vi "API_Edit.vi"(1 "Cancel":bool, 2 "OK":bool, 3 "VI Path":path, 4 "Argument List In":string[](array[string])) -> (0 "Argument List Out":string[](array[string]))   [LabVIEW 2011]
doc: "This VI handles the event loop for API VI's in \"Edit Mode\". Note that the calling VI must have \"OK\" and \"Cancel\" buttons, with labels set as such. This VI also handles window modes for the calling API VI. This VI should always be used in conjunction with API_Init.vi.\n\nThe \"OK\" and \"Cancel\" parameters are optional. They are only necessary if the user wishes to implement their own edit mode event loop in the API VI. In this case, \"OK\" should be set to \"True\" if the user wishes to save the front panel controls in the \"Argument List\". Otherwise, \"Cancel\" should be set to \"True\". If neither of these parameters are set, this VI will handle the edit mode event loop itself."
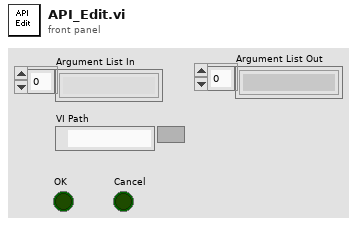
[diagram p1: front panel]
types:
  T1 = enum32{"Invalid", "Default", "Floating", "Floating/Auto-Hide", "Modal"}
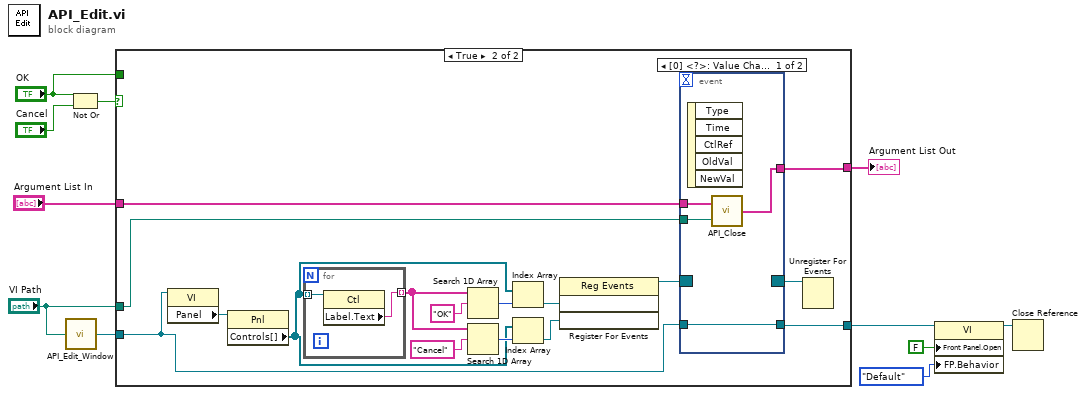
[diagram p0: block diagram]
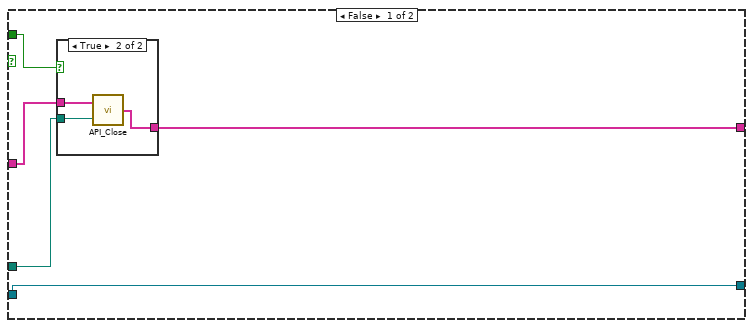
[diagram p2: hidden frame]
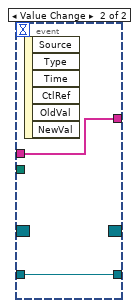
[diagram p4: hidden frame]
diagram:
  n1 = call "API_Edit_Window.vi"("VI Path"="VI Path") -> ("VI Reference"=w1:refnum<vi>)
  n2 = Not Or(1:"Cancel", 2:"OK") -> (0:w4:bool)
  n3 = case shown="True" w4 {
    tunnel: "Argument List In" -> [w14 w26]
    tunnel: "VI Path" -> [w13 w25]
    tunnel: [w12 w24] -> w9
    tunnel: [w16 w23] -> w8
    tunnel: w1 -> [w16 w21]
    tunnel: "OK" -> [w15 _]
    frame False {
      n4 = case shown="True" w15 {
        tunnel: w14 -> [w17 w20]
        tunnel: w13 -> [_ w19]
        tunnel: [w17 w18] -> w12
        frame False {
        }
        frame True {
          n5 = call "API_Close.vi"("VI Path"=w19, "Argument List In"=w20) -> ("Argument List Out"=w18:string[])
        }
      }
    }
    frame True {
      n6 = property class="VI"(reference=w21) -> ("Panel"=w36:refnum<vi>)  [unwired: 1 in, 2 out]
      n7 = property class="Pnl"(reference=w36) -> ("Controls[]"=w30:refnum<vi>[])  [unwired: 1 in, 2 out]
      n8 = for {
        tunnel: w30 -> [w44] mode=indexing
        tunnel: [w43] -> w33 mode=indexing
        n9 = property class="Ctl"(reference=w44) -> ("Label.Text"=w43:string)  [unwired: 1 in, 2 out]
      }
      n10 = Search 1D Array(1D array=w33, element="OK") -> (index of element=w32:i32)  [unwired: 1 in]
      n11 = Search 1D Array(1D array=w33, element="Cancel") -> (index of element=w31:i32)  [unwired: 1 in]
      n12 = Index Array(array=w30, index=w32) -> (element=w29:refnum<vi>)
      n13 = Index Array(array=w30, index=w31) -> (element=w27:refnum<vi>)
      n14 = register-events(w29, w27) -> (reference out=w28:refnum<event-registration>)  [unwired: 2 in, 1 out]
      n15 = event shown="[0] <?>: Value Change" {
        selector: w28 -> [_ _]
        dyn-events: [_ _] -> w22
        timeout: _ -> [_ _]
        tunnel: w26 -> [w39 w42]
        tunnel: [w38 w42] -> w24
        tunnel: [w40 w41] -> w23
        tunnel: w21 -> [w40 w41]
        tunnel: w25 -> [w37 _]
        event Value Change {
          n16 = event-data() -> ()  [unwired: 6 out]
          n17 = call "API_Close.vi"("VI Path"=w37, "Argument List In"=w39) -> ("Argument List Out"=w38:string[])
        }
        event Value Change {
          n18 = event-data() -> ()  [unwired: 7 out]
        }
      }
      n19 = Unregister For Events(event registration refnum=w22) -> ()  [unwired: 1 in, 1 out]
    }
  }
  "Argument List Out" <- w9
  n20 = property class="VI"(reference=w8, "Front Panel.Open"=FALSE ("Front Panel Window:Open"), "FP.Behavior"=T1."Default" ("Front Panel Window:Behavior")) -> (reference out=w5:refnum<vi>)  [unwired: 1 in, 1 out]
  n21 = Close Reference(reference=w5) -> ()  [unwired: 1 in, 1 out]
